vi "Read Device Board.vi"(8 "error in (no error)":errorcluster, 11 "Resource in":refnum<class "DeployResource.lvclass">) -> (0 "error out":errorcluster, 2 "Board":string, 3 "Resource out":refnum<class "DeployResource.lvclass">)   [LabVIEW 2020, in "PicoG-Core.lvlib" / "DeployResource.lvclass"]
uses:
  DeployResource.lvclass
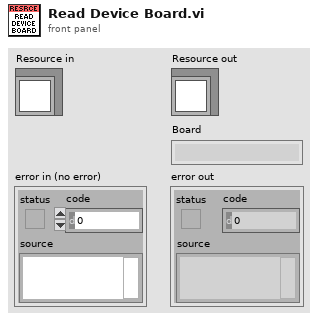
[diagram p1: front panel]
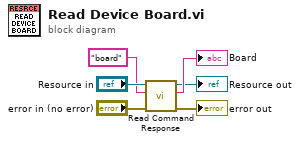
[diagram p0: block diagram]
diagram:
  n1 = call "Read Command Response.vi"("error in (no error)"="error in (no error)", "Shell Command"="board", "Resource in"="Resource in") -> ("error out"=→"error out":errorcluster, "Value"=→"Board":string, "Resource out"=→"Resource out":refnum<class "DeployResource.lvclass">)  [unwired: 6 in]
